vi "Sprachtabelle laden.vi"(11 "Dateipfad (Dialog verwenden)":path) -> (3 "all rows":string[][](array[string]) caption="Alle Zeilen")   [LabVIEW 2015, in "Sprachverwaltung.lvlib"]
uses:
  Sprachverwaltung.lvlib
  <vilib>/Utility/file.llb/Read Delimited Spreadsheet (string).vi
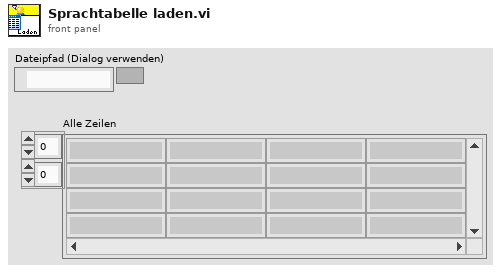
[diagram p1: front panel]
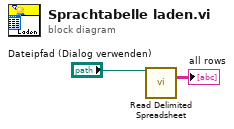
[diagram p0: block diagram]
diagram:
  n1 = call-poly <vilib>:"Read Delimited Spreadsheet.vi"("file path (dialog if empty)"="Dateipfad (Dialog verwenden)") -> ("all rows"=→"all rows":string[][])  [unwired: 9 in, 5 out]
